vi "INDIVIDUAL_VALVE_SET.vi"(8 "Input Value":bool, 10 "Channel ID IN":i32=-999999, 11 "DAQmx Global Channel IN":refnum<k21>) -> ()   [LabVIEW 2013]
doc: "Actually interfaces with the hardware to set a valve value. Originally this was intended to invert certain channels, but that functionality has been disabled."
uses:
  <vilib>/DAQmx/write.llb/DAQmx Write (Digital Bool 1Line 1Point).vi
  <vilib>/DAQmx/miscellaneous.llb/DAQmx Fill In Error Info.vi
panel:
  # "This subVI is somewhat unnecessary now, since\nnone of the valve channels are inverted anymore."
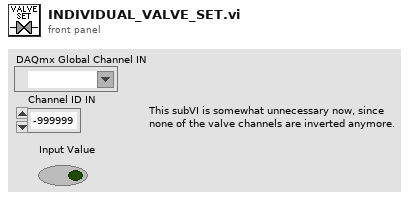
[diagram p1: front panel]
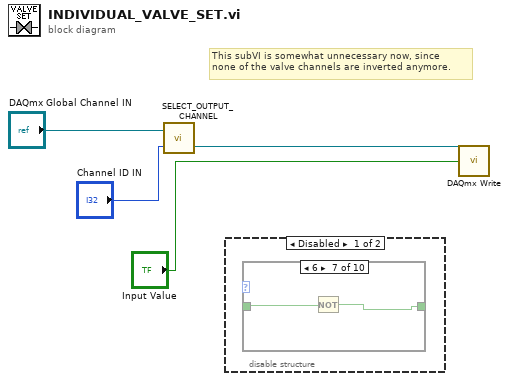
[diagram p0: block diagram]
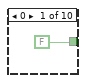
[diagram p2: hidden frame]
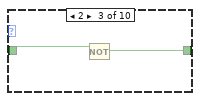
[diagram p4: hidden frame]
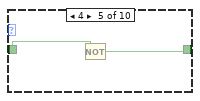
[diagram p6: hidden frame]
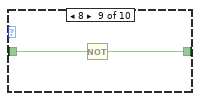
[diagram p9: hidden frame]
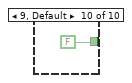
[diagram p10: hidden frame]
diagram:
  # "This subVI is somewhat unnecessary now, since\nnone of the valve channels are inverted anymore."
  n1 = call "SELECT_OUTPUT_CHANNEL.vi"("Channel ID IN"="Channel ID IN", "DAQmx Global Channel IN"="DAQmx Global Channel IN") -> ("DAQmx Global Channel OUT"=w2:refnum<k21>)  [unwired: 1 out]
  n2 = disable-structure shown="Disabled" {
    frame Disabled {
      n3 = case shown="6" {
        selector: _ -> [_ _ _ _ _ _ _ _ _ _]
        tunnel: _ -> [_ w6 w8 w9 w11 w12 w14 w15 w17 _]
        tunnel: [FALSE w6 w7 w9 w10 w12 w13 w15 w16 FALSE] -> _
        frame 0 {
        }
        frame 1 {
        }
        frame 2 {
          n4 = Not(x=w8) -> (.not. x?=w7:bool)
        }
        frame 3 {
        }
        frame 4 {
          n5 = Not(x=w11) -> (.not. x?=w10:bool)
        }
        frame 5 {
        }
        frame 6 {
          n6 = Not(x=w14) -> (.not. x?=w13:bool)
        }
        frame 7 {
        }
        frame 8 {
          n7 = Not(x=w17) -> (.not. x?=w16:bool)
        }
        frame 9, Default {
        }
      }
    }
    frame Enabled {
    }
  }
  n8 = call-poly <vilib>:"DAQmx Write.vi"("task/channels in"=w2, "data"="Input Value") -> ()  [unwired: 11 in, 3 out]
